vi "GetParam.vi"(8 "error in (no error)":errorcluster caption="entrée d'erreur (pas d'erreur)", 11 "MinMaxScaler.lvclass":refnum<class "MinMaxScaler.lvclass">) -> (0 "error out":errorcluster caption="sortie d'erreur", 2 "MinMaxScaler":T1={"feature_range"={"min"=0.0, "max"=1.0}, "copy"=TRUE}, 3 "MinMaxScaler.lvclass":refnum<class "MinMaxScaler.lvclass">)   [LabVIEW 2020, in "MinMaxScaler.lvclass"]
doc: "Get Parameters"
uses:
  MinMaxScaler.lvclass
  MinMaxScaler.lvclass/MinMaxScaler.ctl
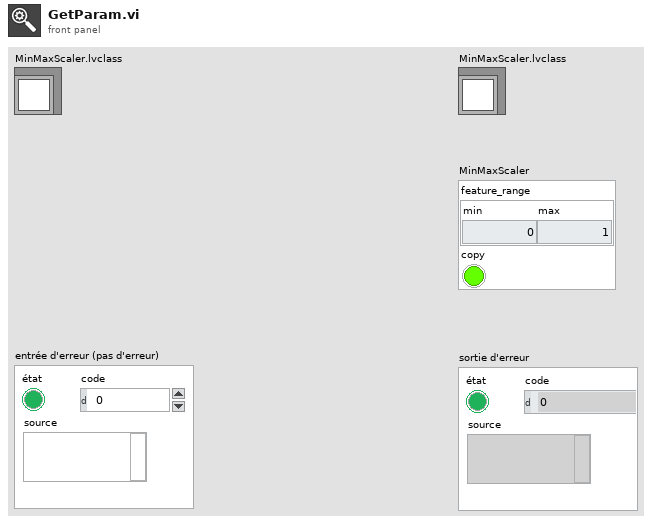
[diagram p1: front panel]
types:
  T1 = cluster{"feature_range":cluster{"min":dbl, "max":dbl}, "copy":bool}
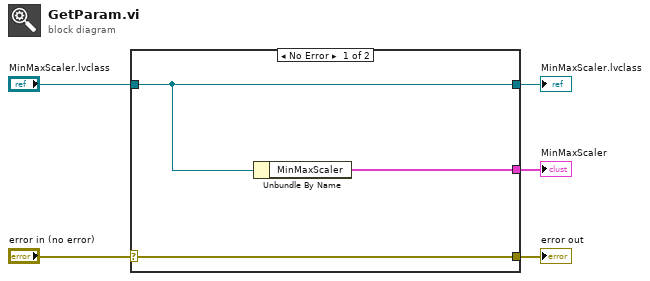
[diagram p0: block diagram]
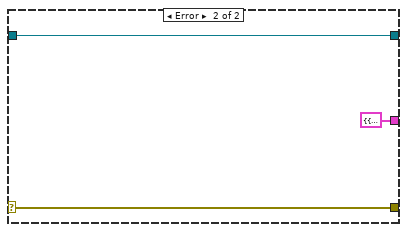
[diagram p2: hidden frame]
diagram:
  n1 = case shown="No Error" "error in (no error)" {
    selector: "error in (no error)" -> [w8 w10]
    tunnel: [w8 w10] -> w4
    tunnel: [w7 w11] -> w2
    tunnel: "MinMaxScaler.lvclass" -> [w7 w11]
    tunnel: [w6 T1 {"feature_range"={"min"=0.0, "max"=0.0}, "copy"=FALSE} ("MinMaxScaler")] -> w1
    frame No Error {
      n2 = Unbundle By Name(w7) -> ("MinMaxScaler"=w6:T1)
    }
    frame Error {
    }
  }
  "error out" <- w4
  "MinMaxScaler.lvclass" <- w2
  "MinMaxScaler" <- w1
